vi "Set RFmx VNA Session.vi"(0 "TSM Context":T1, 5 "VST Instrument Name":string, 7 "RFmx VNA Session":refnum<k21>, 11 "error in":errorcluster) -> (15 "error out":errorcluster)   [LabVIEW 2023, in "RFCalAndFixtureCharact.Common.lvlib"]
uses:
  RFCalAndFixtureCharact.Common.lvlib
  <vilib>/NI_TestStand_SemiconductorModule/NI_TestStand_Semiconductor_Module.lvlibp/PinMap/General/SemiconductorModuleContext.ctl
  Global Data Id Prefix.vi
  <vilib>/NI_TestStand_SemiconductorModule/NI_TestStand_Semiconductor_Module.lvlibp
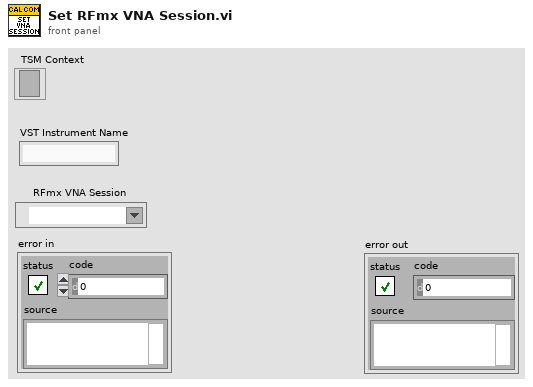
[diagram p1: front panel]
types:
  T1 = typedef "NI_TestStand_Semiconductor_Module.lvlibp/SemiconductorModuleContext.ctl" = refnum<k7>
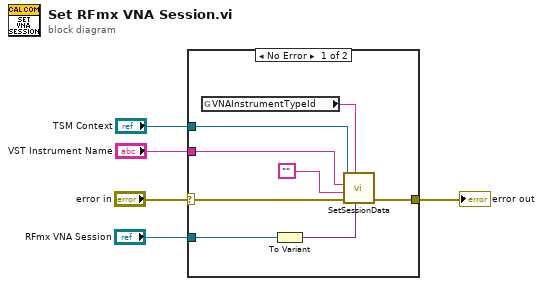
[diagram p0: block diagram]
diagram:
  n1 = case shown="No Error" "error in" {
    selector: "error in" -> [w6 w14]
    tunnel: "TSM Context" -> [w13 _]
    tunnel: "VST Instrument Name" -> [w12 _]
    tunnel: [w9 w14] -> w3
    tunnel: "RFmx VNA Session" -> [w8 _]
    frame No Error {
      n2 = global read "Global Data Id Prefix.vi" "VNAInstrumentTypeId"() -> (w11:string)
      n3 = To Variant(anything=w8) -> (Variant=w7:variant)
      n4 = call <vilib>:"SetSessionData.vi"("Session Data"=w7, "Instrument Type Id"=w11, "error in (no error)"=w6, "Channel Group Id"="", "Instrument Name"=w12, "Semiconductor Module Context"=w13) -> ("error out"=w9:errorcluster)  [unwired: 4 in, 1 out]
    }
    frame Error {
    }
  }
  "error out" <- w3
